vi "PathPlanner_PathFinder_TopKey.vi"() -> (0 "Found":bool, 1 "DoublePair":T2, 3 "PathPlannerFinderGridPosition":T1)   [LabVIEW 2019, in "PathPlanner24.lvlib"]
uses:
  TypeDef/PathPlannerFinderDoublePair.ctl
  PathPlanner_GridPosition_Get.vi
  PathPlanner24.lvlib
  PathPlanner_PathFinder_Globals.vi
  TypeDef/PathPlannerFinderGridPosition.ctl
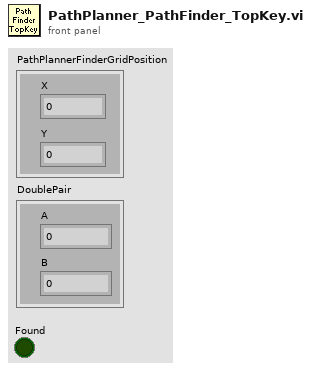
[diagram p1: front panel]
types:
  T1 = typedef "PathPlanner24.lvlib/PathPlannerFinderGridPosition.ctl" = cluster{"X":i32, "Y":i32}
  T2 = typedef "PathPlanner24.lvlib/PathPlannerFinderDoublePair.ctl" = cluster{"A":dbl, "B":dbl}
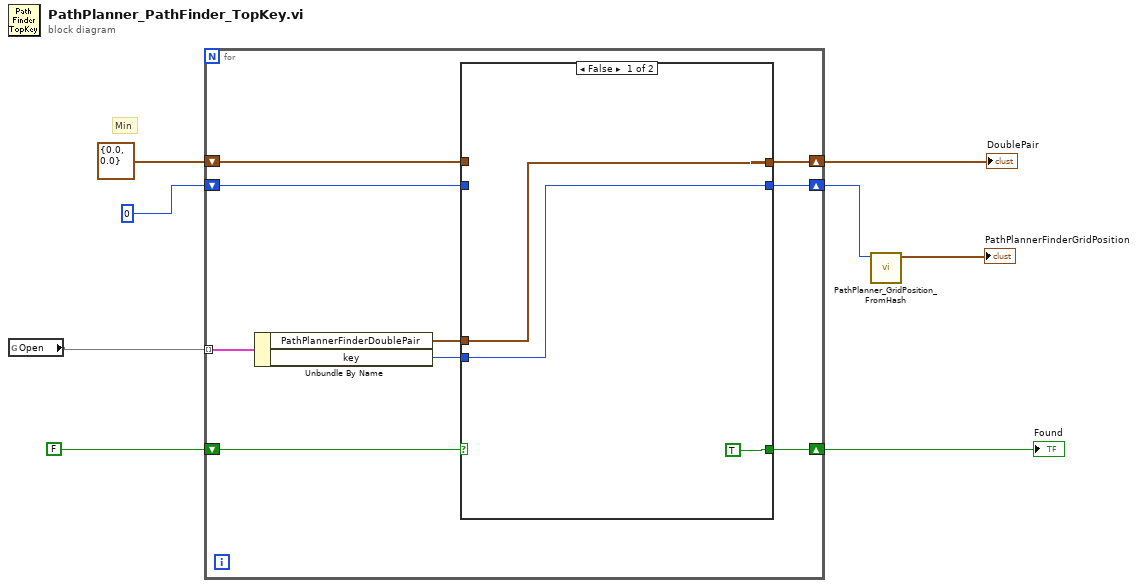
[diagram p0: block diagram]
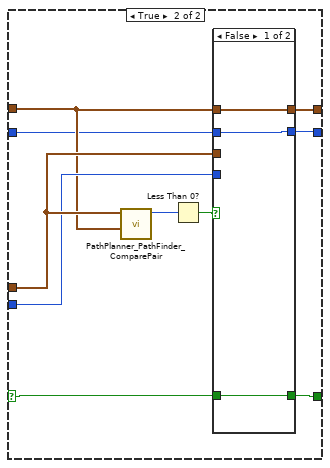
[diagram p2: hidden frame]
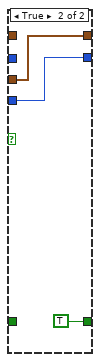
[diagram p3: hidden frame]
diagram:
  # "Min"
  n1 = global read "PathPlanner_PathFinder_Globals.vi" "Open"() -> (w8:map{i32, T2})
  n2 = for {
    tunnel: w8 -> [w16] mode=indexing
    shift-right: [w11] -> w6
    shift-left: FALSE -> [w17]
    shift-right: [w15] -> w4
    shift-left: T2 {"A"=0.0, "B"=0.0} ("DoublePair") -> [w10]
    shift-right: [w13] -> w2
    shift-left: 0 ("key") -> [w9]
    n3 = Unbundle By Name(w16) -> ("PathPlannerFinderDoublePair"=w14:T2, "key"=w12:i32)
    n4 = case shown="False" w17 {
      selector: w17 -> [_ w21]
      tunnel: [w20 w28] -> w15
      tunnel: w14 -> [w20 w27]
      tunnel: [w19 w26] -> w13
      tunnel: w12 -> [w19 w25]
      tunnel: [TRUE w22] -> w11
      tunnel: w10 -> [_ w24]
      tunnel: w9 -> [_ w23]
      frame False {
      }
      frame True {
        n5 = call "PathPlanner_PathFinder_ComparePair.vi"("B"=w24, "A"=w27) -> ("Compare"=w30:i32)  [unwired: 9 in]
        n6 = Less Than 0?(x=w30) -> (x < 0?=w29:bool)
        n7 = case shown="False" w29 {
          tunnel: [w33 w36] -> w28
          tunnel: w27 -> [_ w36]
          tunnel: [w32 w35] -> w26
          tunnel: w25 -> [_ w35]
          tunnel: w24 -> [w33 _]
          tunnel: w23 -> [w32 _]
          tunnel: [w31 TRUE] -> w22
          tunnel: w21 -> [w31 _]
          frame False {
          }
          frame True {
          }
        }
      }
    }
  }
  "DoublePair" <- w4
  "Found" <- w6
  n8 = call "PathPlanner_GridPosition_FromHash.vi"("Hash"=w2) -> ("GridPosition"=→"PathPlannerFinderGridPosition":T1)  [unwired: 10 in]
